vi "Set Value.vi"(8 "error in":errorcluster, 10 "Image":variant[][](array[variant]), 11 "Selection Views in":refnum<class "Graph with Section Views.lvclass">) -> (0 "error out":errorcluster, 3 "Selection Views out":refnum<class "Graph with Section Views.lvclass">)   [LabVIEW 2025, in "Graph with Section Views.lvclass"]
uses:
  Graph with Section Views.lvclass
  Base Graph/Base Graph.lvclass/Base Graph.ctl
  Graph with Section Views.lvclass/Graph with Section Views.ctl
  Base Graph/Base Graph.lvclass
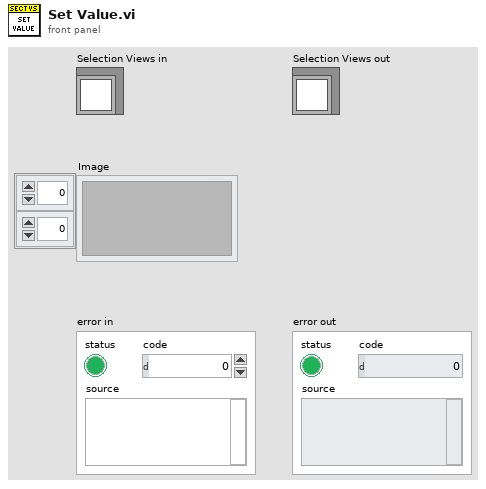
[diagram p1: front panel]
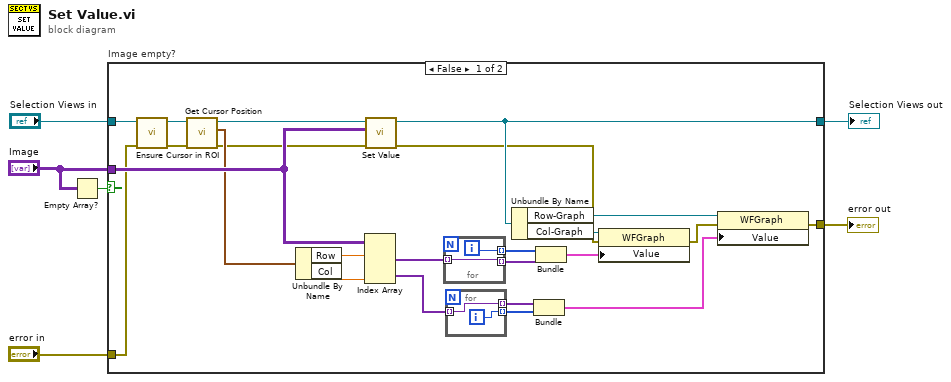
[diagram p0: block diagram]
diagram:
  n1 = Empty Array?(array="Image") -> (empty?=w4:bool)
  n2 = case "Image empty?" shown="False" w4 {
    tunnel: [w18 w35] -> w5
    tunnel: "Selection Views in" -> [w8 w35]
    tunnel: "Image" -> [w17 _]
    tunnel: [w15 w34] -> w2
    tunnel: "error in" -> [w12 w34]
    frame False {
      n3 = call "Ensure Cursor in ROI.vi"("error in"=w12, "Base Graph in"=w8) -> ("error out"=w11:errorcluster, "Base Graph out"=w7:refnum<class "Graph with Section Views.lvclass">)  [unwired: 8 in]
      n4 = call "Get Cursor Position.vi"("Base Graph in"=w7) -> ("Cursor Position"=w16:cluster{"Col":dbl, "Row":dbl}, "Base Graph out"=w19:refnum<class "Graph with Section Views.lvclass">)  [unwired: 9 in]
      n5 = Unbundle By Name(w16) -> ("Row"=w29:dbl, "Col"=w10:dbl)
      n6 = Index Array(array=w17, index (row) #1=w29, index (col) #2=w10) -> (element #1=w21:variant[], element #2=w9:variant[])  [unwired: 2 in]
      n7 = call-parent "Set Value.vi"("error in"=w11, "Image"=w17, "Base Graph in"=w19) -> ("error out"=w13:errorcluster, "Base Graph out"=w18:refnum<class "Graph with Section Views.lvclass">)  [unwired: 7 in]
      n8 = for {
        tunnel: [w30] -> w23 mode=indexing
        tunnel: w21 -> [w31] mode=indexing
        tunnel: [w31] -> w20 mode=indexing
        i -> [w30]
      }
      n9 = for {
        tunnel: [w32] -> w28 mode=indexing
        tunnel: w9 -> [w33] mode=indexing
        tunnel: [w33] -> w22 mode=indexing
        i -> [w32]
      }
      n10 = Unbundle By Name(w18) -> ("Row-Graph"=w27:refnum<vi>, "Col-Graph"=w26:refnum<vi>)
      n11 = Bundle(w22, w28) -> (w24:cluster{variant[], i32[]})  [unwired: 1 in]
      n12 = Bundle(w23, w20) -> (w25:cluster{i32[], variant[]})  [unwired: 1 in]
      n13 = property class="WFGraph"(reference=w26, error in=w13, "Value"=w25) -> (error out=w14:errorcluster)  [unwired: 1 out]
      n14 = property class="WFGraph"(reference=w27, error in=w14, "Value"=w24) -> (error out=w15:errorcluster)  [unwired: 1 out]
    }
    frame True {
    }
  }
  "Selection Views out" <- w5
  "error out" <- w2
